vi "get randomized team.vi"(9 "# of Teams":i32, 10 "u":i32, 11 "Flag Array":bool[][](array[boolean])) -> (2 "This Team":i32)   [LabVIEW 2013]
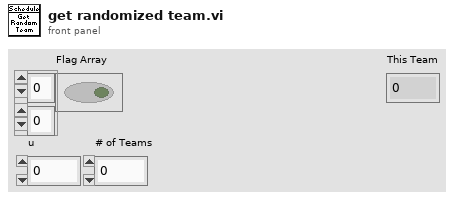
[diagram p1: front panel]
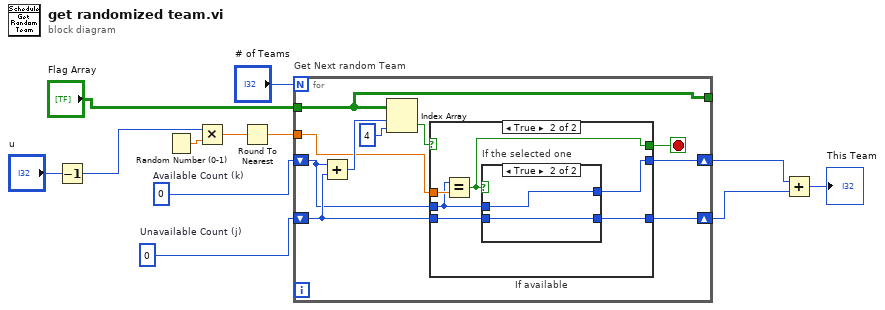
[diagram p0: block diagram]
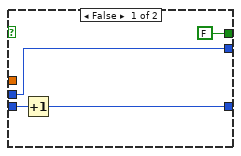
[diagram p2: hidden frame]
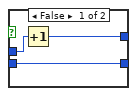
[diagram p3: hidden frame]
diagram:
  w10 = 0  # Unavailable Count (j)
  w11 = 0  # Available Count (k)
  n1 = Decrement(x="u") -> (x-1=w6:i32)
  n2 = Random Number (0-1)() -> (number: 0 to 1=w12:dbl)
  n3 = Multiply(x=w6, y=w12) -> (x*y=w8:dbl)
  n4 = Round To Nearest(number=w8) -> (nearest integer value=w9:dbl)
  n5 = for "Get Next random Team" {
    N: "# of Teams" -> [_]
    tunnel: "Flag Array" -> [w13]
    shift-right: [w16] -> w4
    shift-left: w11 -> [w17]
    shift-right: [w18] -> w3
    shift-left: w10 -> [w19]
    tunnel: w9 -> [w15]
    tunnel: [w13] -> _
    stop <- w14 stop-if-true
    n6 = Add(x=w17, y=w19) -> (x+y=w22:i32)
    n7 = Index Array(array=w13, index (row)=w22, index (col)=4 ("disabled index (col)")) -> (element=w20:bool)
    n8 = case "If available" shown="True" w20 {
      tunnel: w19 -> [w26 w29]
      tunnel: [w25 w27] -> w18
      tunnel: w17 -> [w24 w30]
      tunnel: [w24 w28] -> w16
      tunnel: w15 -> [_ w32]
      tunnel: [FALSE w31] -> w14
      frame False {
        n9 = Increment(x=w26) -> (x+1=w25:i32)
      }
      frame True {
        n10 = Equal?(x=w30, y=w32) -> (x = y?=w31:bool)
        n11 = case "If the selected one" shown="True" w31 {
          tunnel: w30 -> [w35 w37]
          tunnel: [w34 w37] -> w28
          tunnel: w29 -> [w33 w36]
          tunnel: [w33 w36] -> w27
          frame False {
            n12 = Increment(x=w35) -> (x+1=w34:i32)
          }
          frame True {
          }
        }
      }
    }
  }
  n13 = Add(x=w4, y=w3) -> (x+y=→"This Team":i32)
